vi "PID Performance Evaluation.vi"(6 "reinitialize? (F)":bool, 7 "output":dbl format="%.2f", 8 "dt (s)":dbl=-1.0 format="%.3f", 9 "cost type":u16(ring) items=["Integral Error (IE)", "Integral Absolute Error (IAE)", "Integral Square Error (ISE)", "Integral Time Absolute Error (ITAE)", "Integral Time Error (ITE)", "Integral Time Square Error (ITSE)", "Integral Square Time Error (ISTE)"], 10 "process variable":dbl format="%.2f", 11 "setpoint":dbl format="%.2f") -> (3 "Cost":dbl)   [LabVIEW 2020, in "NI_PID_autopid.lvlib"]
uses:
  <vilib>/addons/control/pid/NI_PID_autopid.lvlib
  <vilib>/addons/control/pid/NI_PID_pid.lvlib
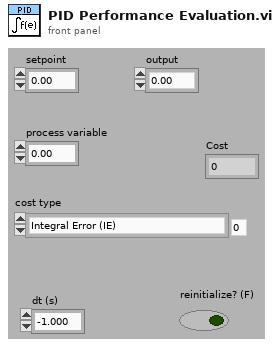
[diagram p1: front panel]
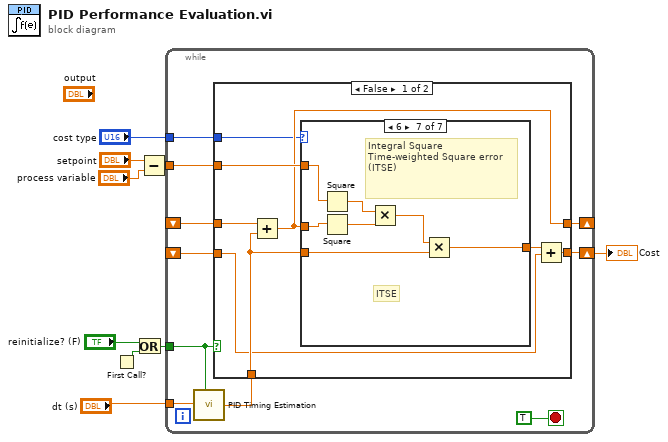
[diagram p0: block diagram]
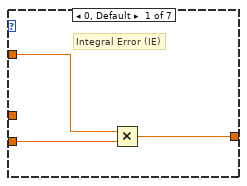
[diagram p2: hidden frame]
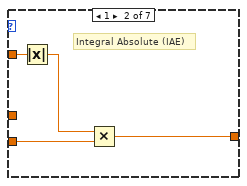
[diagram p3: hidden frame]
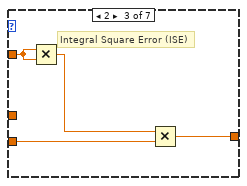
[diagram p4: hidden frame]
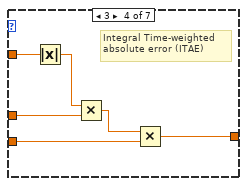
[diagram p5: hidden frame]
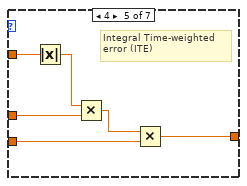
[diagram p6: hidden frame]
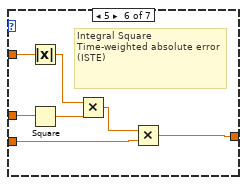
[diagram p7: hidden frame]
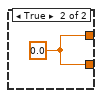
[diagram p8: hidden frame]
diagram:
  n1 = First Call?() -> (First Call?: T/F=w7:bool)
  n2 = Or(x="reinitialize? (F)", y=w7) -> (x .or. y?=w6:bool)
  n3 = Subtract(x="setpoint", y="process variable") -> (x-y=w2:dbl)
  n4 = while {
    tunnel: w2 -> [w19]
    tunnel: "dt (s)" -> [w13]
    tunnel: w6 -> [w11]
    shift-right: [w18] -> w5
    shift-left: _ -> [w16]
    shift-right: [w15] -> _
    shift-left: _ -> [w14]
    tunnel: "cost type" -> [w10]
    stop <- TRUE stop-if-true
    n5 = call <vilib>:"PID Timing Estimation.vi"("Initialize?"=w11, "dt (s) in"=w13) -> ("dt (s) out"=w12:dbl)  [unwired: 7 in]
    n6 = case shown="False" w11 {
      tunnel: w19 -> [w27 _]
      tunnel: [w26 w65] -> w18
      tunnel: w12 -> [w24 _]
      tunnel: w16 -> [w21 _]
      tunnel: [w22 w65] -> w15
      tunnel: w14 -> [w23 _]
      tunnel: w10 -> [w20 _]
      frame False {
        n7 = Add(x=w23, y=w24) -> (x+y=w22:dbl)
        n8 = case shown="6" w20 {
          tunnel: w27 -> [w29 w33 w37 w42 w48 w55 w62]
          tunnel: w24 -> [w30 w34 w38 w40 w46 w53 w60]
          tunnel: w22 -> [_ _ _ w41 w47 w54 w61]
          tunnel: [w28 w32 w35 w39 w45 w51 w58] -> w25
          frame 0, Default {
            # "Integral Error (IE)"
            n9 = Multiply(x=w29, y=w30) -> (x*y=w28:dbl)
          }
          frame 1 {
            # "Integral Absolute (IAE)"
            n10 = Absolute Value(x=w33) -> (abs(x)=w31:dbl)
            n11 = Multiply(x=w31, y=w34) -> (x*y=w32:dbl)
          }
          frame 2 {
            # "Integral Square Error (ISE)"
            n12 = Multiply(x=w37, y=w37) -> (x*y=w36:dbl)
            n13 = Multiply(x=w36, y=w38) -> (x*y=w35:dbl)
          }
          frame 3 {
            # "Integral Time-weighted \nabsolute error (ITAE)"
            n14 = Absolute Value(x=w42) -> (abs(x)=w44:dbl)
            n15 = Multiply(x=w44, y=w41) -> (x*y=w43:dbl)
            n16 = Multiply(x=w43, y=w40) -> (x*y=w39:dbl)
          }
          frame 4 {
            # "Integral Time-weighted \nerror (ITE)"
            n17 = Absolute Value(x=w48) -> (abs(x)=w50:dbl)
            n18 = Multiply(x=w50, y=w47) -> (x*y=w49:dbl)
            n19 = Multiply(x=w49, y=w46) -> (x*y=w45:dbl)
          }
          frame 5 {
            # "Integral Square Time-weighted absolute error (ISTE)"
            n20 = Absolute Value(x=w55) -> (abs(x)=w57:dbl)
            n21 = Square(x=w54) -> (x^2=w52:dbl)
            n22 = Multiply(x=w57, y=w52) -> (x*y=w56:dbl)
            n23 = Multiply(x=w56, y=w53) -> (x*y=w51:dbl)
          }
          frame 6 {
            # "Integral Square Time-weighted Square error (ITSE)"
            # "ITSE"
            n24 = Square(x=w62) -> (x^2=w64:dbl)
            n25 = Square(x=w61) -> (x^2=w59:dbl)
            n26 = Multiply(x=w64, y=w59) -> (x*y=w63:dbl)
            n27 = Multiply(x=w63, y=w60) -> (x*y=w58:dbl)
          }
        }
        n28 = Add(x=w25, y=w21) -> (x+y=w26:dbl)
      }
      frame True {
        w65 = 0.0
      }
    }
  }
  "Cost" <- w5
